vi "MsgBox_LV.vi"(8 "Error in":errorcluster caption="Error in (no error)", 9 "timeout (ms)":i32=3000, 10 "strCaption":string, 11 "strText":string) -> (0 "Error out":errorcluster)   [LabVIEW 2013]
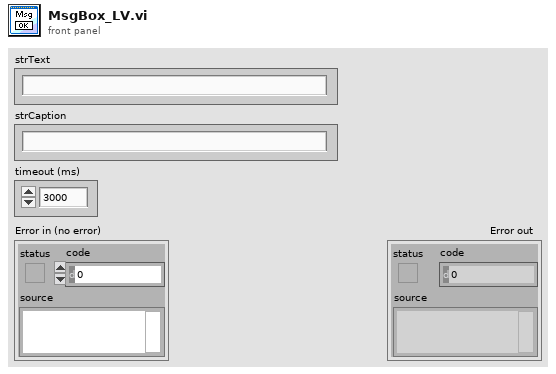
[diagram p1: front panel]
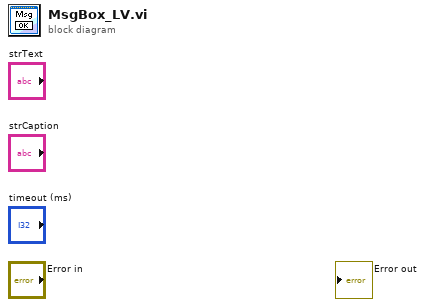
[diagram p0: block diagram]
diagram:
